vi "N1.vi"() -> ()   [LabVIEW 2020]
panel:
  out "Answer":dbl
  out "Error":string
  in  "Numeric":dbl
  in  "?":bool
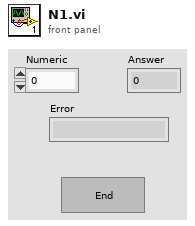
[diagram p1: front panel]
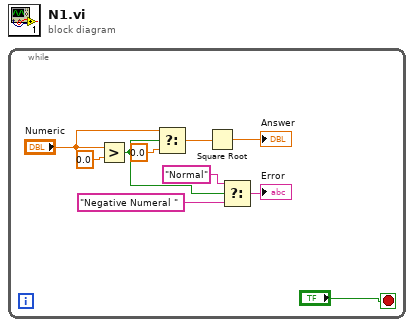
[diagram p0: block diagram]
diagram:
  n1 = while {
    stop <- "?" stop-if-true
    n2 = Greater?(x="Numeric", y=0.0) -> (0:w7:bool)
    n3 = Select(t="Numeric", s=w7, f=0.0) -> (s? t:f=w4:dbl)
    n4 = Square Root(x=w4) -> (sqrt(x)=→"Answer":dbl)
    n5 = Select(t="Normal", s=w7, f="Negative Numeral ") -> (s? t:f=→"Error":string)
  }
